vi "Read Duration.vi"(8 "error in (no error)":errorcluster, 11 "TimedDirector in":refnum<class "TimedDirector.lvclass">) -> (0 "error out":errorcluster, 2 "Duration":u32 caption="ms" step=1 format="%.0g", 3 "TimedDirector out":refnum<class "TimedDirector.lvclass">)   [LabVIEW 2023, in "HAF.lvlib" / "TimedDirector.lvclass"]
uses:
  TimedDirector.lvclass
  TimedDirector.lvclass/TimedDirector.ctl
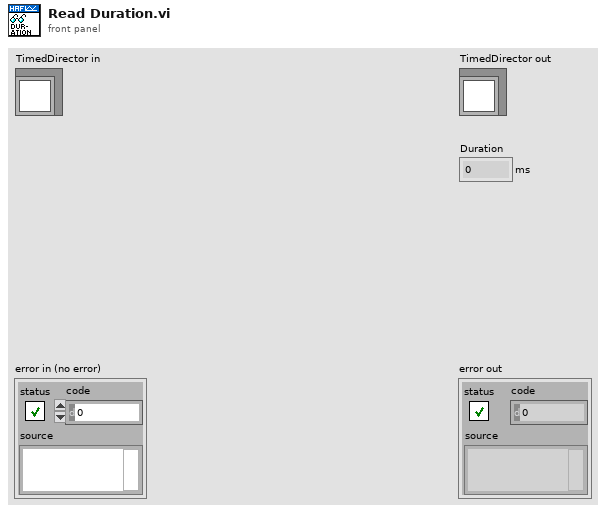
[diagram p1: front panel]
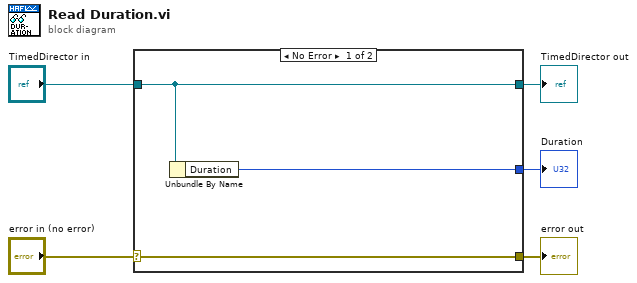
[diagram p0: block diagram]
diagram:
  n1 = case shown="No Error" "error in (no error)" {
    selector: "error in (no error)" -> [w8 w9]
    tunnel: [w8 w9] -> w4
    tunnel: [w7 w10] -> w2
    tunnel: "TimedDirector in" -> [w7 w10]
    tunnel: [w6 _] -> w1
    frame No Error {
      n2 = Unbundle By Name(w7) -> ("Duration"=w6:u32)
    }
    frame Error {
    }
  }
  "error out" <- w4
  "TimedDirector out" <- w2
  "Duration" <- w1
